vi "specialUrlEncode.vi"(11 "str":string) -> (3 "UrlEncode":string)   [LabVIEW 2016]
uses:
  System.Web
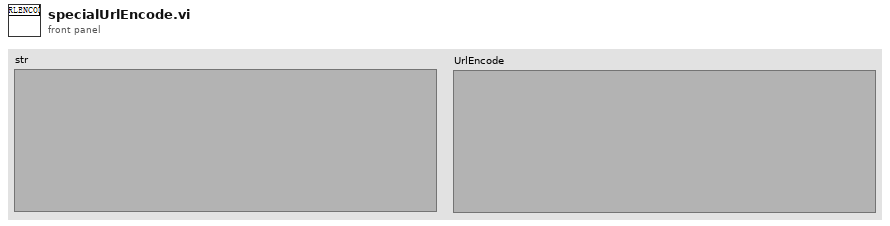
[diagram p1: front panel]
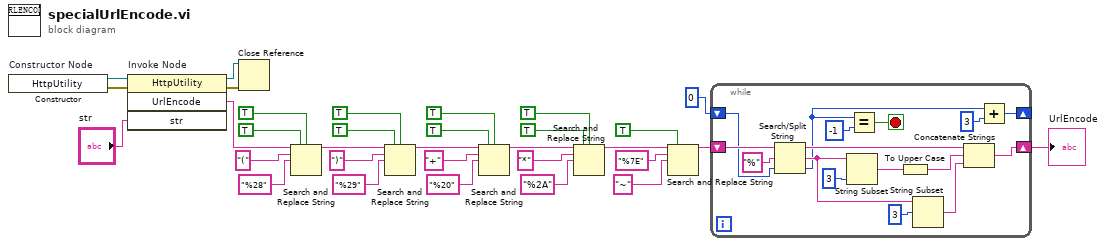
[diagram p0: block diagram]
diagram:
  n1 = constructor on="Constructor Node" class="HttpUtility"() -> (reference out=w32:refnum<k24>, error out=w31:errorcluster)  [unwired: 3 in, 1 out]
  n2 = invoke on="Invoke Node" class="HttpUtility" method="UrlEncode"(reference=w32, error in=w31, "str"="str") -> (reference out=w29:refnum<k24>, error out=w30:errorcluster, "UrlEncode"=w8:string)  [unwired: 1 in, 1 out]
  n3 = Close Reference(reference=w29, error in (no error)=w30) -> ()  [unwired: 1 out]
  n4 = Search and Replace String(replace all?=TRUE ("替换全部？(F)"), case sensitive?=TRUE ("忽略大小写？(F)"), input string=w8, search string="(" ("搜索字符串"), replace string="%28" ("替换字符串(\"\")")) -> (result string=w3:string)  [unwired: 3 in, 3 out]
  n5 = Search and Replace String(replace all?=TRUE ("替换全部？(F)"), case sensitive?=TRUE ("忽略大小写？(F)"), input string=w3, search string=")" ("搜索字符串"), replace string="%29" ("替换字符串(\"\")")) -> (result string=w1:string)  [unwired: 3 in, 3 out]
  n6 = Search and Replace String(replace all?=TRUE ("替换全部？(F)"), case sensitive?=TRUE ("忽略大小写？(F)"), input string=w1, search string="+" ("搜索字符串"), replace string="%20" ("替换字符串(\"\")")) -> (result string=w14:string)  [unwired: 3 in, 3 out]
  n7 = Search and Replace String(replace all?=TRUE ("替换全部？(F)"), case sensitive?=TRUE ("忽略大小写？(F)"), input string=w14, search string="*" ("搜索字符串"), replace string="%2A" ("替换字符串(\"\")")) -> (result string=w23:string)  [unwired: 3 in, 3 out]
  n8 = Search and Replace String(replace all?=TRUE ("替换全部？(F)"), input string=w23, search string="%7E" ("搜索字符串"), replace string="~" ("替换字符串(\"\")")) -> (result string=w17:string)  [unwired: 4 in, 3 out]
  n9 = while {
    shift-right: [w38] -> w18
    shift-left: w17 -> [w48]
    shift-right: [w44] -> _
    shift-left: 0 -> [w46]
    stop <- w35 stop-if-true
    n10 = Search/Split String(string=w48, search string/char (-)="%" ("搜索字符串/字符(-)"), offset (0)=w46) -> (substring before match=w40:string, match + rest of string=w42:string, offset of match=w37:i32)
    n11 = String Subset(string=w42, length (rest)=3 ("长度（剩余）")) -> (substring=w34:string)  [unwired: 1 in]
    n12 = Equal?(x=w37, y=-1) -> (x = y?=w35:bool)
    n13 = To Upper Case(1:w34) -> (0:w33:string)
    n14 = String Subset(string=w42, offset (0)=3 ("偏移量(0)")) -> (substring=w39:string)  [unwired: 1 in]
    n15 = Concatenate Strings(w40, w33, w39) -> (w38:string)
    n16 = Add(x=w37, y=3) -> (x+y=w44:i32)
  }
  "UrlEncode" <- w18
